vi "Drive Immediate.vi"(7 "Description":string, 8 "Command Info In":T1, 9 "Fly wheel":dbl, 10 "Launcher":dbl, 11 "Intake":dbl) -> (0 "Command Info Out":T1)   [LabVIEW 2018]
doc: "Often used for joystick control, this VI checks to see that the joystick axes are outside the deadband and updates the motors appropriately."
uses:
  <vilib>/Rock Robotics/WPI/Framework/Command Status Info.ctl
  <vilib>/Rock Robotics/WPI/Framework/Completion Status.ctl
  <vilib>/Rock Robotics/WPI/Framework/Completion Notifier.ctl
  Implementation/Drive Setpoints.ctl
  Implementation/Drive Operations.ctl
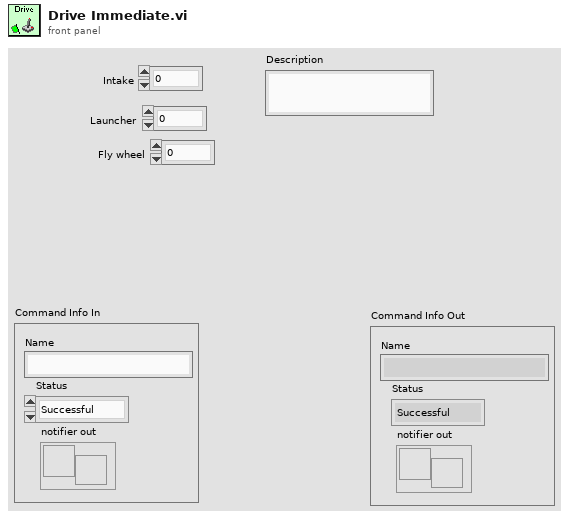
[diagram p1: front panel]
types:
  T1 = typedef "Command Status Info.ctl" = cluster{"Name":string, "Status":T2, "notifier out":T3}
  T2 = typedef "Completion Status.ctl" = enum16{"Successful", "Aborted", "Incomplete"}
  T3 = typedef "Completion Notifier.ctl" = refnum<notifier>
  T4 = typedef "Drive Setpoints.ctl" = cluster{"Operation":T5, "Intake speed":dbl, "Duration":dbl, "Flywheel":dbl, "Launcher":dbl}
  T5 = typedef "Drive Operations.ctl" = enum16{"Reserve", "Read Current", "Immediate", "Drive for Time", "Drive for Distance"}
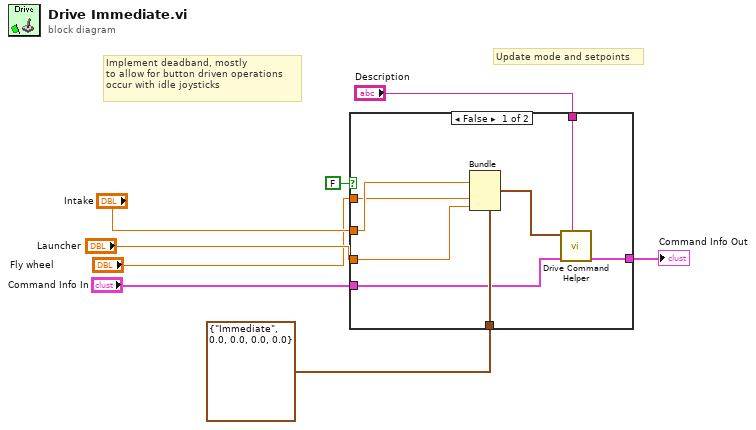
[diagram p0: block diagram]
diagram:
  # "Implement deadband, mostly\nto allow for button driven operations\noccur with idle joysticks"
  # "Update mode and setpoints"
  n1 = case shown="False" FALSE {
    tunnel: "Intake" -> [w11 _]
    tunnel: T4 {"Operation"=enum."Immediate", "Intake speed"=0.0, "Duration"=0.0, "Flywheel"=0.0, "Launcher"=0.0} ("SubSystem Data") -> [w16 _]
    tunnel: [w15 w17] -> w8
    tunnel: "Command Info In" -> [w14 w17]
    tunnel: "Description" -> [w12 _]
    tunnel: "Launcher" -> [w10 _]
    tunnel: "Fly wheel" -> [w9 _]
    frame False {
      n2 = Bundle(cluster=w16, "Intake speed"=w11, "Flywheel"=w9, "Launcher"=w10) -> (w13:T4)  [unwired: 2 in]
      n3 = call "Drive Command Helper.vi"("Description"=w12, "Command Info In"=w14, "SubSystem Data"=w13) -> ("Command Info Out"=w15:T1)  [unwired: 6 in, 2 out]
    }
    frame True {
    }
  }
  "Command Info Out" <- w8
